vi "NewtonsPSM_WaitData.vi"(6 "error in (no error)":errorcluster, 9 "VISA session":refnum<visa-resource-name>) -> (0 "error out":errorcluster, 2 "Data Available":bool, 3 "dup VISA session":refnum<visa-resource-name>)   [LabVIEW 2025, in "NewtonsPSM1735.lvlib"]
doc: "This VI wait for available data before query a result."
uses:
  NewtonsPSM1735.lvlib
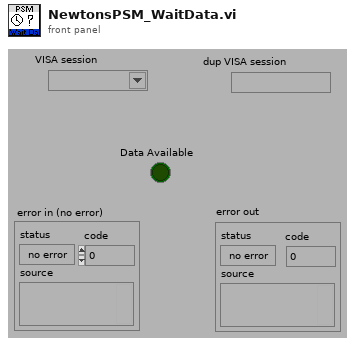
[diagram p1: front panel]
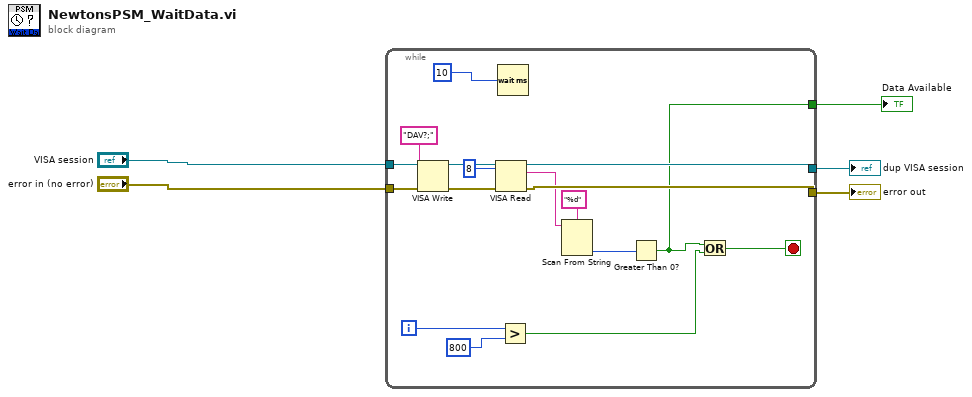
[diagram p0: block diagram]
diagram:
  n1 = while {
    tunnel: "error in (no error)" -> [w22]
    tunnel: [w16] -> w5
    tunnel: "VISA session" -> [w20]
    tunnel: [w17] -> w4
    tunnel: [w9] -> w3
    i -> [w11]
    stop <- w8 stop-if-true
    n2 = VISA Write(VISA resource name=w20, write buffer="DAV?;", error in (no error)=w22) -> (VISA resource name out=w19:refnum<visa-resource-name>, error out=w18:errorcluster)  [unwired: 1 out]
    n3 = VISA Read(VISA resource name=w19, byte count=u32 8 ("nombre d'octets"), error in (no error)=w18) -> (VISA resource name out=w17:refnum<visa-resource-name>, read buffer=w15:string, error out=w16:errorcluster)  [unwired: 1 out]
    n4 = Wait (ms)(milliseconds to wait=10) -> ()  [unwired: 1 out]
    n5 = Greater?(x=w11, y=800) -> (0:w7:bool)
    n6 = Scan From String(format string="%d" ("chaîne de format"), input string=w15) -> (output 1=w13:i32)  [unwired: 2 in, 4 out]
    n7 = Greater Than 0?(x=w13) -> (x > 0?=w9:bool)
    n8 = Or(x=w9, y=w7) -> (x .or. y?=w8:bool)
  }
  "error out" <- w5
  "dup VISA session" <- w4
  "Data Available" <- w3
